vi "stopServer.vi"(8 "error in (no error)":errorcluster, 11 "TcpServerBase in":refnum<class "TcpServerBase.lvclass">) -> (0 "error out":errorcluster, 3 "TcpServerBase out":refnum<class "TcpServerBase.lvclass">)   [LabVIEW 2018, in "TcpServerBase.lvclass"]
doc: "Send a notifier to stop all TCP servers."
uses:
  TcpServerBase.lvclass
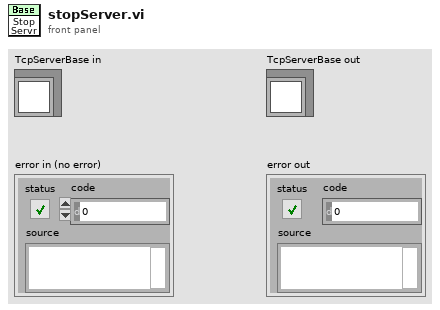
[diagram p1: front panel]
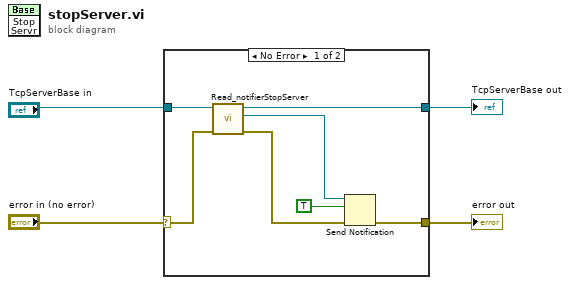
[diagram p0: block diagram]
diagram:
  n1 = case shown="No Error" "error in (no error)" {
    selector: "error in (no error)" -> [w6 w12]
    tunnel: "TcpServerBase in" -> [w8 w13]
    tunnel: [w7 w13] -> w3
    tunnel: [w5 w12] -> w1
    frame No Error {
      n2 = call "Read_notifierStopServer.vi"("error in (no error)"=w6, "TcpServerBase in"=w8) -> ("error out"=w9:errorcluster, "notifierStopServer"=w10:refnum<notifier>, "TcpServerBase out"=w7:refnum<class "TcpServerBase.lvclass">)  [unwired: 7 in]
      n3 = Send Notification(notification=TRUE, notifier=w10, error in (no error)=w9) -> (error out=w5:errorcluster)  [unwired: 1 out]
    }
    frame Error {
    }
  }
  "error out" <- w1
  "TcpServerBase out" <- w3
